vi "is_moving_requested.vi"(8 "error in (no error)":errorcluster, 11 "GenericStage in":refnum<class "GenericStage.lvclass">) -> (0 "error out":errorcluster, 2 "moving requested?":bool, 3 "GenericStage out":refnum<class "GenericStage.lvclass">)   [LabVIEW 2010, in "GenericStage.lvclass"]
uses:
  GenericStage.lvclass
  translation_mode_enum.ctl
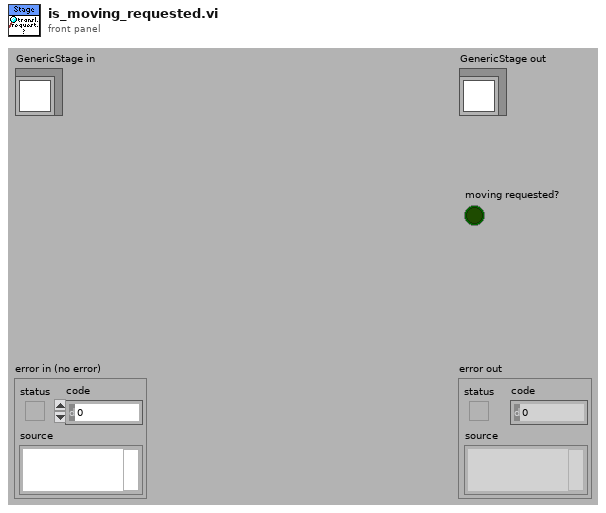
[diagram p1: front panel]
types:
  T1 = typedef "GenericStage.lvclass/translation_mode_enum.ctl" = enum16{"DON'T MOVE", "relative", "absolute"}
  T2 = typedef "GenericStage.lvclass/translation_request.ctl" = cluster{"translation mode":T1, "translation vector":refnum<class "SpaceVector.lvclass">}
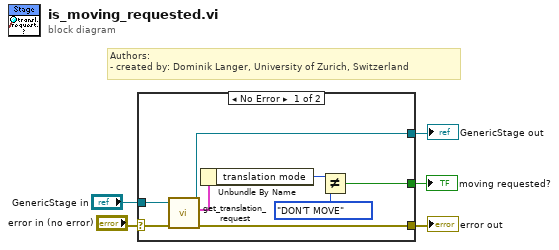
[diagram p0: block diagram]
diagram:
  # "Authors: \n- created by: Dominik Langer, University of Zurich, Switzerland"
  n1 = case shown="No Error" "error in (no error)" {
    selector: "error in (no error)" -> [w13 w15]
    tunnel: [w12 w15] -> w4
    tunnel: [w6 w14] -> w2
    tunnel: "GenericStage in" -> [w7 w14]
    tunnel: [w8 _] -> w1
    frame No Error {
      n2 = call-dynamic "get_translation_request.vi"("error in (no error)"=w13, "GenericStage.lvclass in"=w7) -> ("error out"=w12:errorcluster, "translation request"=w11:T2, "GenericStage.lvclass out"=w6:refnum<class "GenericStage.lvclass">)  [unwired: 7 out]
      n3 = Unbundle By Name(w11) -> ("translation mode"=w10:T1)
      n4 = Not Equal?(x=w10, y=translation_mode_enum."DON'T MOVE") -> (x != y?=w8:bool)
    }
    frame Error {
    }
  }
  "error out" <- w4
  "GenericStage out" <- w2
  "moving requested?" <- w1
